vi "Read Server Stop.vi"(8 "error in":errorcluster, 11 "ServiceBase in":refnum<class "ServiceBase.lvclass">) -> (0 "error out":errorcluster, 2 "Server Stop":refnum<user-event>, 3 "ServiceBase out":refnum<class "ServiceBase.lvclass">)   [LabVIEW 2019, in "gRPC-servicer.lvlib" / "ServiceBase.lvclass"]
uses:
  ServiceBase.lvclass
  ServiceBase.lvclass/ServiceBase.ctl
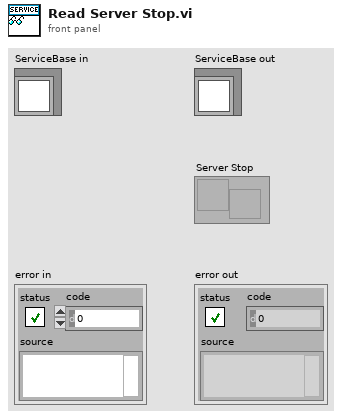
[diagram p1: front panel]
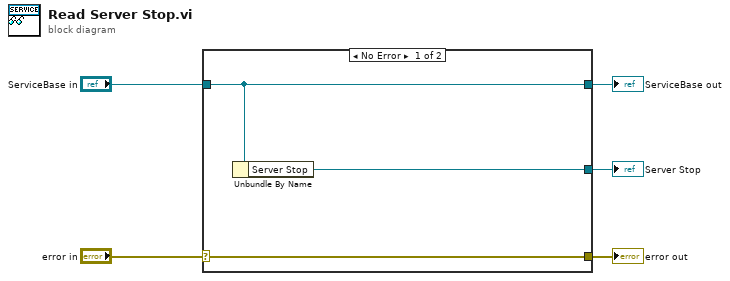
[diagram p0: block diagram]
diagram:
  n1 = case shown="No Error" "error in" {
    selector: "error in" -> [w8 w10]
    tunnel: [w8 w10] -> w4
    tunnel: [w7 w9] -> w2
    tunnel: "ServiceBase in" -> [w7 w9]
    tunnel: [w6 _] -> w1
    frame No Error {
      n2 = Unbundle By Name(w7) -> ("Server Stop"=w6:refnum<user-event>)
    }
    frame Error {
    }
  }
  "error out" <- w4
  "ServiceBase out" <- w2
  "Server Stop" <- w1
